vi "Update UI Display Wrapper.vi"(8 "error in (no error)":errorcluster, 10 "Update for Display":string, 11 "LabVIEW Build Script in":refnum<class "LabVIEW Build Script.lvclass">) -> (0 "error out":errorcluster)   [LabVIEW 2021, in "LabVIEW Build Script.lvclass"]
uses:
  LabVIEW Build Script.lvclass
  LabVIEW Build Script.lvclass/LabVIEW Build Script.ctl
  Build Script Common/Build Script Common.lvlib
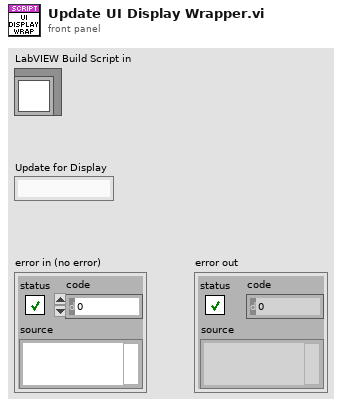
[diagram p1: front panel]
types:
  T1 = typedef "Build Script Common.lvlib/References.ctl" = cluster{"UI Display":refnum<vi>, "UI Display Valid":bool, "UI Semaphore":T2}
  T2 = typedef "Semaphore RefNum" = refnum<k1>
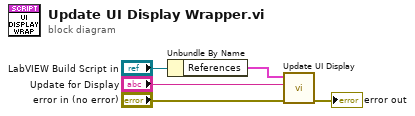
[diagram p0: block diagram]
diagram:
  n1 = Unbundle By Name("LabVIEW Build Script in") -> ("References"=w2:T1)
  n2 = call "Update UI Display.vi"("error in (no error)"="error in (no error)", "Update for Display"="Update for Display", "References"=w2) -> ("error out"=→"error out":errorcluster)  [unwired: 8 in]
